vi "Vol-menu.vi"(8 "error in (no error)":errorcluster, 11 "menu":refnum<k9>) -> (0 "error out":errorcluster, 3 "menu reference out":refnum<k9>)   [LabVIEW 2020]
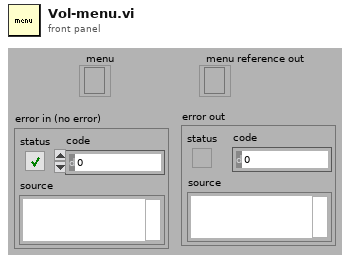
[diagram p1: front panel]
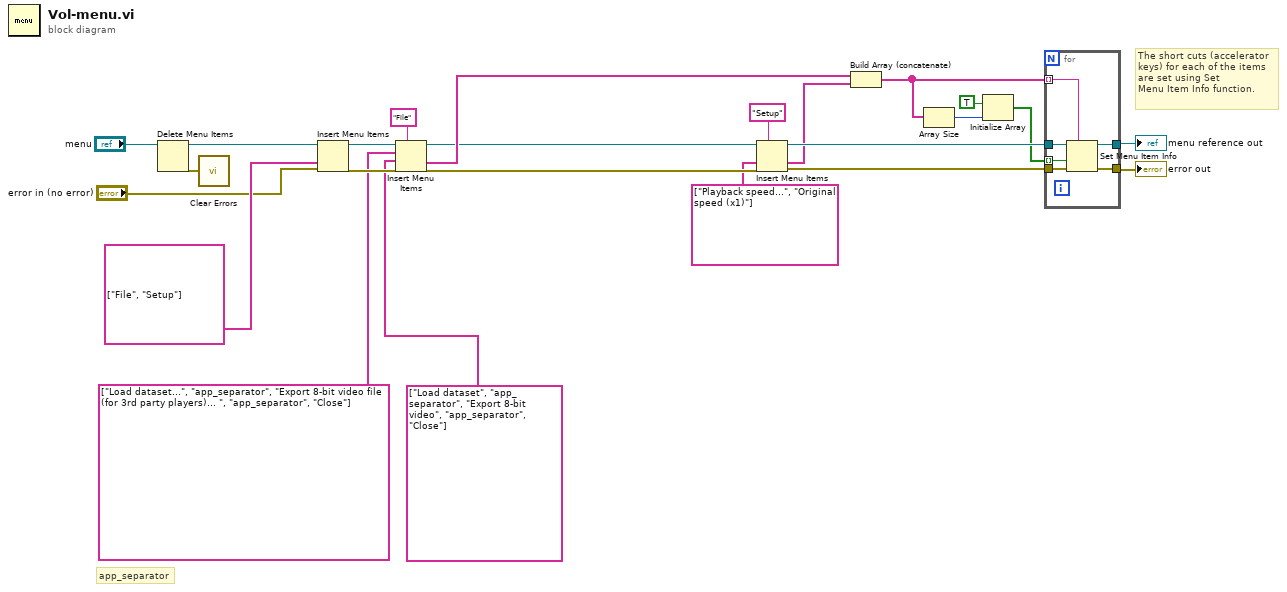
[diagram p0: block diagram]
diagram:
  # "app_separator"
  # "The short cuts (accelerator\nkeys) for each of the items\nare set using Set\nMenu Item Info function."
  n1 = Delete Menu Items(9:"menu") -> (0:w14:errorcluster, 3:w20:refnum<k9>)  [unwired: 2 in, 1 out]
  n2 = call <vilib>:"Clear Errors.vi"("error in (no error)"=w14) -> ()  [unwired: 5 in, 2 out]
  n3 = Insert Menu Items(6:"error in (no error)", 7:string[] ["File", "Setup"] ("item tags"), 9:w20) -> (0:w22:errorcluster, 3:w15:refnum<k9>)  [unwired: 4 out]
  n4 = Insert Menu Items(5:"File" ("menu tag"), 6:w22, 7:string[] ["Load dataset", "app_separator", "Export 8-bit video", "app_separator", "Close"] ("item tags"), 8:string[] ["Load dataset...", "app_separator", "Export 8-bit video file (for 3rd party players)... ", "app_separator", "Close"] ("item tags"), 9:w15) -> (0:w23:errorcluster, 1:w19:string[], 3:w16:refnum<k9>)  [unwired: 1 out]
  n5 = Insert Menu Items(5:"Setup" ("menu tag"), 6:w23, 7:string[] ["Playback speed...", "Original speed (x1)"] ("item tags"), 9:w16) -> (0:w12:errorcluster, 1:w10:string[], 3:w11:refnum<k9>)  [unwired: 2 out]
  n6 = Build Array (concatenate)(w19, w10) -> (w7:string[])
  n7 = Array Size(array=w7) -> (size(s)=w9:i32)
  n8 = Initialize Array(TRUE, w9) -> (w8:bool[])
  n9 = for {
    tunnel: w11 -> [w30]
    tunnel: [w29] -> w18
    tunnel: w7 -> [w28] mode=indexing
    tunnel: w12 -> [w27]
    tunnel: [w26] -> w24
    tunnel: w8 -> [w25] mode=indexing
    n10 = Set Menu Item Info(7:w28, 8:w27, 9:w25, 11:w30) -> (0:w26:errorcluster, 3:w29:refnum<k9>)  [unwired: 1 in, 2 out]
  }
  "error out" <- w24
  "menu reference out" <- w18
